vi "Begin.vi"(11 "Image Size":T1=enum."160x120") -> (0 "error out":errorcluster)   [LabVIEW 2011]
doc: "Called before other user functions, this VI is expected to open initial I/O refnums, load in file data, and do all program initialization. Notice that the <B>error out</B> terminal is simply used for data flow. Wiring it to other structures or subVIs ensures that this VI runs first."
uses:
  <vilib>/Rock Robotics/WPI/Camera/WPI_CameraImageSize.ctl
  <vilib>/Rock Robotics/WPI/Joystick/WPI_JoystickDeviceEnum.ctl
  <vilib>/Rock Robotics/SystemInterfaces/DIO/FPGA_DIOPWMChannel.ctl
  <vilib>/Rock Robotics/WPI/RobotDrive/WPI_RobotDriveOpen4MotorWithJaguar.vi
  <vilib>/Rock Robotics/WPI/Camera/WPI_CameraWhite Balance Values.ctl
  <vilib>/Rock Robotics/WPI/Camera/WPI_CameraExposure Values.ctl
  <vilib>/Rock Robotics/WPI/Camera/WPI_CameraFrameRate.ctl
  <vilib>/Rock Robotics/WPI/Relay/WPI_RelayDirection.ctl
  <vilib>/Rock Robotics/SystemInterfaces/Typedef/FPGA_TypedefDigitalModule.ctl
  <vilib>/Rock Robotics/SystemInterfaces/DIO/FPGA_DIORelayChannel.ctl
  <vilib>/Rock Robotics/WPI/MotorControl/WPI_MotorControlOpen Victor.vi
  <vilib>/Rock Robotics/SystemInterfaces/DIO/FPGA_DIOChannel.ctl
  <vilib>/Rock Robotics/WPI/MotorControl/WPI_MotorControlOpen Jaguar.vi
  <vilib>/Rock Robotics/WPI/Counter/WPI_CounterDigitalInputToDigitalSource.vi
  <vilib>/Rock Robotics/WPI/Encoder/WPI_EncoderType.ctl
  <vilib>/Rock Robotics/SystemInterfaces/AI/FPGA_AIGyroChannel.ctl
  <vilib>/Rock Robotics/SystemInterfaces/AI/FPGA_AIChannel.ctl
  <vilib>/Rock Robotics/WPI/MotorControl/WPI_MotorControlOpenCANJaguar.vi
  <vilib>/Rock Robotics/WPI/CAN/Jaguar/SubVIs/WPI_CANJaguar_ControlMode.ctl
  <vilib>/Rock Robotics/WPI/CAN/Jaguar/SubVIs/WPI_CANJaguar_SpeedReference.ctl
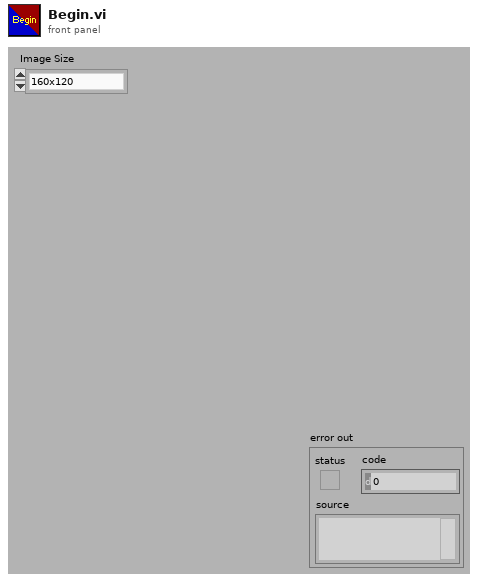
[diagram p1: front panel]
types:
  T1 = typedef "WPI_CameraImageSize.ctl" = enum16{"640x480", "320x240", "160x120"}
  T2 = typedef "FPGA_DIOPWMChannel.ctl" = enum8{"PWM 1", "PWM 2", "PWM 3", "PWM 4", "PWM 5", "PWM 6", "PWM 7", "PWM 8", "PWM 9", "PWM 10", "Invalid"}
  T3 = typedef "WPI_JoystickDeviceEnum.ctl" = enum16{"USB 1", "USB 2", "USB 3", "USB 4", "Kinect 1", "Kinect 2"}
  T4 = typedef "WPI_CameraFrameRate.ctl" = u32
  T5 = typedef "WPI_CameraExposure Values.ctl" = enum16{"Auto", "Flicker-free 50 Hz", "Flicker-free 60 Hz", "Hold current"}
  T6 = typedef "WPI_CameraWhite Balance Values.ctl" = enum16{"Auto", "Fixed indoor", "Fixed outdoor 1", "Fixed outdoor 2", "Fixed fluorescent 1", "Fixed fluorescent 2", "Hold current"}
  T7 = typedef "WPI_CameraDevRef.ctl" = cluster{"Camera Address":string, "CameraStatus":errorcluster, "Acquire Image Notifier":refnum<notifier>}
  T8 = typedef "FPGA_AIGyroChannel.ctl" = enum8{"AI 1", "AI 2", "Invalid"}
  T9 = typedef "WPI_GyroDevRef.ctl" = cluster{"DevStatus":errorcluster, "Analog Module":T10, "Analog Channel":T11, "Offset":dbl, "Gain (VoltsPerDegree/Second)":dbl}
  T10 = typedef "FPGA_TypedefAnalogModule.ctl" = enum16{"Analog Module 1", "Analog Module 2"}
  T11 = typedef "FPGA_AIChannel.ctl" = enum8{"AI 1", "AI 2", "AI 3", "AI 4", "AI 5", "AI 6", "AI 7", "AI 8", "Invalid"}
  T12 = typedef "FPGA_TypedefDigitalModule.ctl" = enum16{"Digital Module 1", "Digital Module 2"}
  T13 = typedef "WPI_CANJaguar_ControlMode.ctl" = enum8{"Percent VBus", "Current", "Speed", "Position", "Voltage"}
  T14 = typedef "WPI_MotorControlDeviceRef.ctl" = cluster{"DeviceStatus":errorcluster, "Type":enum16{"PWM", "CAN"}, "PWM":cluster{"Digital Module":T12, "PWM Channel":T2, "DeadBand":T15}, "CAN":cluster{"Device Number":u8, "Control Mode":T13, "Semaphore":T16, "Max Vout":dbl}, "Invert":bool, "TransformRef":T17, "InvTransformRef":T17}
  T15 = typedef "WPI_PWMDeadband.ctl" = cluster{"Name":string, "maxPositivePwm":i32, "minPositivePwm":i32, "centerPwm":i32, "maxNegativePwm":i32, "minNegativePwm":i32, "angularRange":u16}
  T16 = typedef "Semaphore RefNum" = refnum<k1>
  T17 = typedef "WPI_PWMTransform_ConPane.ctl" = refnum<vi>
  T18 = typedef "WPI_CANJaguar_SpeedReference.ctl" = u8
  T19 = typedef "FPGA_DIOChannel.ctl" = enum8{"DIO 1", "DIO 2", "DIO 3", "DIO 4", "DIO 5", "DIO 6", "DIO 7", "DIO 8", "DIO 9", "DIO 10", "DIO 11", "DIO 12", "DIO 13", "DIO 14", "Invalid"}
  T20 = typedef "WPI_DigitalInputDevRef.ctl" = cluster{"DevStatus":errorcluster, "DIO Channel":T19, "Digital Module":T12}
  T21 = typedef "WPI_EncoderType.ctl" = enum16{"1x", "2x", "4x"}
  T22 = typedef "FPGA_CounterEncoderSourceConvertionLVSourceType.ctl" = cluster{"DevStatus":errorcluster, "AnalogTriggerMode?":bool, "DigitalMode":cluster{"Digital Module":T12, "DIO Channel":T23}, "AnalogTriggerMode":cluster{"AnalogTriggerIndex":T24, "OutputType":T25}}
  T23 = typedef "FPGA_DIODigitalSourceChannel.ctl" = enum8{"DIO 1", "DIO 2", "DIO 3", "DIO 4", "DIO 5", "DIO 6", "DIO 7", "DIO 8", "DIO 9", "DIO 10", "DIO 11", "DIO 12", "DIO 13", "DIO 14", "Disabled"}
  T24 = typedef "FPGA_AnalogTriggerIndex.ctl" = enum8{"Trig 0", "Trig 1", "Trig 2", "Trig 3", "Trig 4", "Trig 5", "Trig 6", "Trig 7", "Invalid"}
  T25 = typedef "FPGA_AnalogTriggerOutType.ctl" = enum16{"InWindow", "TriggerState", "Rising", "Falling"}
  T26 = typedef "WPI_EncoderDevRef.ctl" = cluster{"DevStatus":errorcluster, "EncoderIndex":T27, "CounterIndex":T28, "DistancePerCount":dbl, "Decoding Type":T21}
  T27 = typedef "FPGA_EncoderIdx.ctl" = enum8{"Enc 0", "Enc 1", "Enc 2", "Enc 3", "Invalid"}
  T28 = typedef "FPGA_CounterCtrSystemIndex.ctl" = enum8{"Ctr 0", "Ctr 1", "Ctr 2", "Ctr 3", "Ctr 4", "Ctr 5", "Ctr 6", "Ctr 7", "Invalid"}
  T29 = typedef "WPI_ServoDeviceRef.ctl" = cluster{"DeviceStatus":errorcluster, "Digital Module":T12, "PWM Channel":T2, "DeadBand":T15}
  T30 = typedef "WPI_AnalogChannelDevRef.ctl" = cluster{"DevStatus":errorcluster, "Analog Module":T10, "Analog Channel":T11}
  T31 = typedef "FPGA_DIORelayChannel.ctl" = enum8{"Relay 1", "Relay 2", "Relay 3", "Relay 4", "Relay 5", "Relay 6", "Relay 7", "Relay 8", "Invalid"}
  T32 = typedef "WPI_RelayDirection.ctl" = enum16{"Both directions", "Forward only", "Reverse only"}
  T33 = typedef "WPI_RelayDevRef.ctl" = cluster{"DevStatus":errorcluster, "Relay Channel":T31, "Digital Module":T12, "Relay Direction":T32}
  T34 = typedef "WPI_RobotDriveDevRef.ctl" = cluster{"DevStatus":errorcluster, "Motors[]":T14[], "Square Inputs":bool, "Max Output":dbl, "Isochronous":bool}
  T35 = typedef "WPI_JoystickDevRef.ctl" = cluster{"Device":T3}
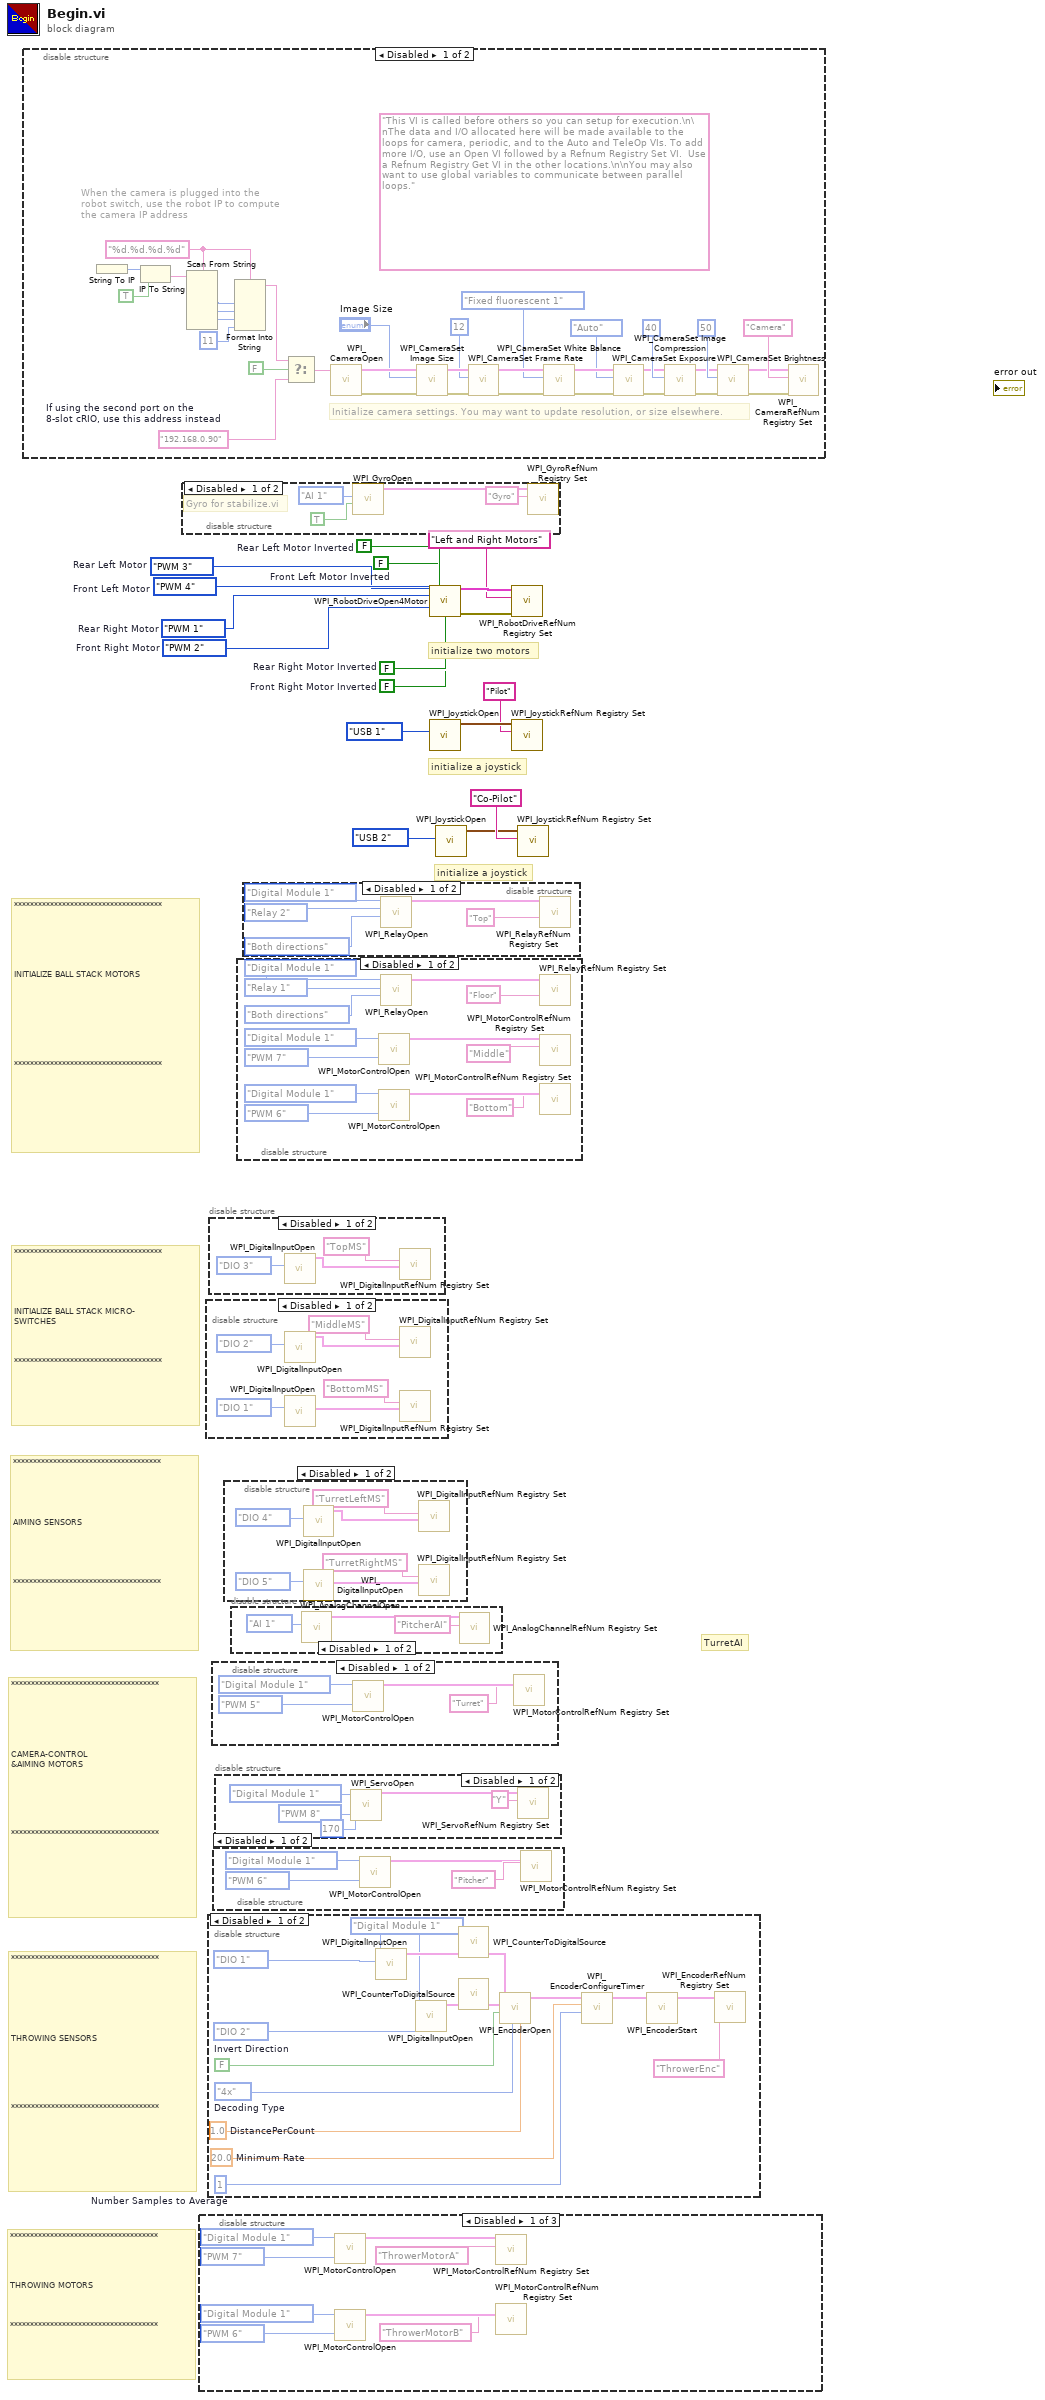
[diagram p0: block diagram]
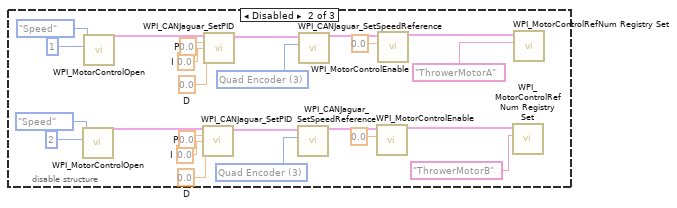
[diagram p13: hidden frame]
diagram:
  w1 = FALSE  # Front Right Motor Inverted
  w2 = FALSE  # Front Left Motor Inverted
  w3 = FPGA_DIOPWMChannel."PWM 3"  # Rear Left Motor
  w4 = FPGA_DIOPWMChannel."PWM 1"  # Rear Right Motor
  w5 = FPGA_DIOPWMChannel."PWM 2"  # Front Right Motor
  w6 = FPGA_DIOPWMChannel."PWM 4"  # Front Left Motor
  w16 = FALSE  # Rear Left Motor Inverted
  w17 = FALSE  # Rear Right Motor Inverted
  # "TurretAI"
  # "*************************************\n\n\n\n\nTHROWING MOTORS\n\n\n\n*************************************"
  # "*************************************\n\n\n\n\n\n\n\nTHROWING SENSORS\n\n\n\n\n\n\n*************************************"
  # "*************************************\n\n\n\n\n\n\nCAMERA-CONTROL\n&AIMING MOTORS\n\n\n\n\n\n\n*************************************"
  # "*************************************\n\n\n\n\n\nAIMING SENSORS\n\n\n\n\n\n*************************************"
  # "*************************************\n\n\n\n\n\nINITIALIZE BALL STACK MICRO-\nSWITCHES\n\n\n\n*************************************"
  # "*************************************\n\n\n\n\n\n\nINITIALIZE BALL STACK MOTORS\n\n\n\n\n\n\n\n\n*************************************"
  # "initialize a joystick"
  # "initialize a joystick"
  # "initialize two motors"
  n1 = disable-structure shown="Disabled" {
    frame Disabled {
      w22 = "%d.%d.%d.%d" ("format string")
      (unwired) "This VI is called before others so you can setup for execution.\n\nThe data and I/O allocated here will be made available to the loops for camera, periodic, and to the Auto and TeleOp VIs. To add more I/O, use an Open VI followed by a Refnum Registry Set VI.  Use a Refnum Registry Get VI in the other locations.\n\nYou may also want to use global variables to communicate between parallel loops."
      w19 = "192.168.0.90"  # If using the second port on the 8-slot cRIO, use this address instead
      # "When the camera is plugged into the\nrobot switch, use the robot IP to compute\nthe camera IP address"
      # "Initialize camera settings. You may want to update resolution, or size elsewhere."
      n2 = String To IP() -> (0:w29:u32)  [unwired: 1 in]
      n3 = IP To String(1:TRUE ("dot notation? (F)"), 2:w29) -> (0:w27:string)
      n4 = Scan From String(format string=w22, input string=w27) -> (output 1=w26:i32, output 2=w25:i32, output 3=w24:i32)  [unwired: 7 in, 3 out]
      n5 = Format Into String(format string=w22, w26, w25, w24, 11 ("Compression")) -> (resulting string=w20:string)  [unwired: 2 in, 1 out]
      n6 = Select(t=w20, s=FALSE, f=w19) -> (s? t:f=w21:string)
      n7 = call <vilib>:"WPI_CameraOpen.vi"("Camera Address"=w21) -> ("error out"=w41:errorcluster, "CameraDevRef"=w42:T7)  [unwired: 1 in, 8 out]
      n8 = call <vilib>:"WPI_CameraSet Image Size.vi"("error in (no error)"=w41, "Image Size"="Image Size", "CameraDevRef"=w42) -> ("error out"=w40:errorcluster, "CameraDevRef Out"=w43:T7)  [unwired: 7 out]
      n9 = call <vilib>:"WPI_CameraSet Frame Rate.vi"("error in (no error)"=w40, "Frame Rate (fps)"=T4 12, "CameraDevRef"=w43) -> ("error out"=w39:errorcluster, "CameraDevRef Out"=w45:T7)  [unwired: 7 out]
      n10 = call <vilib>:"WPI_CameraSet White Balance.vi"("error in (no error)"=w39, "White Balance"=WPI_CameraWhite_Balance_Values."Fixed fluorescent 1", "CameraDevRef"=w45) -> ("error out"=w38:errorcluster, "CameraDevRef Out"=w44:T7)  [unwired: 7 out]
      n11 = call <vilib>:"WPI_CameraSet Exposure.vi"("error in (no error)"=w38, "Exposure"=WPI_CameraExposure_Values."Auto", "CameraDevRef"=w44) -> ("error out"=w37:errorcluster, "CameraDevRef Out"=w47:T7)  [unwired: 7 out]
      n12 = call <vilib>:"WPI_CameraSet Image Compression.vi"("error in (no error)"=w37, "Compression"=40, "CameraDevRef"=w47) -> ("error out"=w36:errorcluster, "CameraDevRef Out"=w46:T7)  [unwired: 7 out]
      n13 = call <vilib>:"WPI_CameraSet Brightness.vi"("error in (no error)"=w36, "Brightness"=50, "CameraDevRef"=w46) -> ("error out"=w34:errorcluster, "CameraDevRef Out"=w35:T7)  [unwired: 7 out]
      n14 = call <vilib>:"WPI_CameraRefNum Registry Set.vi"("error in (no error)"=w34, "refnum name"="Camera", "CameraDevRef"=w35) -> ()  [unwired: 9 out]
    }
    frame Enabled {
    }
  }
  n15 = disable-structure shown="Disabled" {
    frame Disabled {
      # "Gyro for stabilize.vi"
      n16 = call <vilib>:"WPI_GyroOpen.vi"("Calibrate On Open"=TRUE, "Analog Channel"=FPGA_AIGyroChannel."AI 1") -> ("GyroDevRef"=w54:T9)  [unwired: 7 in, 2 out]
      n17 = call <vilib>:"WPI_GyroRefNum Registry Set.vi"("refnum name"="Gyro", "GyroDevRef"=w54) -> ()  [unwired: 8 in, 2 out]
    }
    frame Enabled {
    }
  }
  n18 = disable-structure shown="Disabled" {
    frame Disabled {
      n19 = call-poly <vilib>:"WPI_MotorControlOpen.vi"("PWM Channel"=FPGA_DIOPWMChannel."PWM 7", "Digital Module (Module 1)"=FPGA_TypedefDigitalModule."Digital Module 1") -> ("MotorControlDeviceRef"=w62:T14)  [unwired: 8 in, 1 out]
      n20 = call-poly <vilib>:"WPI_MotorControlOpen.vi"("PWM Channel"=FPGA_DIOPWMChannel."PWM 6", "Digital Module (Module 1)"=FPGA_TypedefDigitalModule."Digital Module 1") -> ("MotorControlDeviceRef"=w58:T14)  [unwired: 8 in, 1 out]
      n21 = call <vilib>:"WPI_MotorControlRefNum Registry Set.vi"("refnum name"="ThrowerMotorA", "MotorControlDevRef"=w62) -> ()  [unwired: 8 in, 2 out]
      n22 = call <vilib>:"WPI_MotorControlRefNum Registry Set.vi"("refnum name"="ThrowerMotorB", "MotorControlDevRef"=w58) -> ()  [unwired: 8 in, 2 out]
    }
    frame Disabled {
      w75 = 0.0  # D
      w74 = 0.0  # I
      w73 = 0.0  # P
      w70 = T18 3 items=["Encoder"=0, "Inv Encoder"=2, "Quad Encoder"=3, "None"=255] ("Speed Reference")
      w76 = 0.0  # D
      w77 = 0.0  # I
      w78 = 0.0  # P
      w81 = T18 3 items=["Encoder"=0, "Inv Encoder"=2, "Quad Encoder"=3, "None"=255] ("Speed Reference")
      n23 = call-poly <vilib>:"WPI_MotorControlOpen.vi"("Device Number"=u8 2, "Control Mode"=WPI_CANJaguar_ControlMode."Speed") -> ("MotorControlDeviceRef"=w71:T14)  [unwired: 8 in, 1 out]
      n24 = call-poly <vilib>:"WPI_MotorControlOpen.vi"("Device Number"=u8 1, "Control Mode"=WPI_CANJaguar_ControlMode."Speed") -> ("MotorControlDeviceRef"=w80:T14)  [unwired: 8 in, 1 out]
      n25 = call <vilib>:"WPI_CANJaguar_SetPID.vi"("CAN Jaguar Ref"=w71, "P"=w73, "I"=w74, "D"=w75) -> ("CAN Jaguar Ref Out"=w69:T14)  [unwired: 10 in, 1 out]
      n26 = call <vilib>:"WPI_CANJaguar_SetPID.vi"("CAN Jaguar Ref"=w80, "P"=w78, "I"=w77, "D"=w76) -> ("CAN Jaguar Ref Out"=w82:T14)  [unwired: 10 in, 1 out]
      n27 = call <vilib>:"WPI_CANJaguar_SetSpeedReference.vi"("Speed Reference"=w70, "CAN Jaguar Ref"=w69) -> ("CAN Jaguar Ref Out"=w67:T14)  [unwired: 8 in, 1 out]
      n28 = call <vilib>:"WPI_CANJaguar_SetSpeedReference.vi"("Speed Reference"=w81, "CAN Jaguar Ref"=w82) -> ("CAN Jaguar Ref Out"=w84:T14)  [unwired: 8 in, 1 out]
      n29 = call <vilib>:"WPI_MotorControlEnable.vi"("Encoder Initial Position"=0.0, "CAN Jaguar Ref"=w67) -> ("CAN Jaguar Ref Out"=w66:T14)  [unwired: 8 in, 1 out]
      n30 = call <vilib>:"WPI_MotorControlEnable.vi"("Encoder Initial Position"=0.0, "CAN Jaguar Ref"=w84) -> ("CAN Jaguar Ref Out"=w85:T14)  [unwired: 8 in, 1 out]
      n31 = call <vilib>:"WPI_MotorControlRefNum Registry Set.vi"("refnum name"="ThrowerMotorB", "MotorControlDevRef"=w66) -> ()  [unwired: 8 in, 2 out]
      n32 = call <vilib>:"WPI_MotorControlRefNum Registry Set.vi"("refnum name"="ThrowerMotorA", "MotorControlDevRef"=w85) -> ()  [unwired: 8 in, 2 out]
    }
    frame Enabled {
    }
  }
  n33 = disable-structure shown="Disabled" {
    frame Disabled {
      n34 = call <vilib>:"WPI_DigitalInputOpen.vi"("DIO Channel"=FPGA_DIOChannel."DIO 2") -> ("DigitalInputDevRef"=w87:T20)  [unwired: 9 in, 1 out]
      n35 = call <vilib>:"WPI_DigitalInputOpen.vi"("DIO Channel"=FPGA_DIOChannel."DIO 1") -> ("DigitalInputDevRef"=w90:T20)  [unwired: 9 in, 1 out]
      n36 = call <vilib>:"WPI_DigitalInputRefNum Registry Set.vi"("refnum name"="MiddleMS", "DigitalInputDevRef"=w87) -> ()  [unwired: 8 in, 2 out]
      n37 = call <vilib>:"WPI_DigitalInputRefNum Registry Set.vi"("refnum name"="BottomMS", "DigitalInputDevRef"=w90) -> ()  [unwired: 8 in, 2 out]
    }
    frame Enabled {
    }
  }
  n38 = disable-structure shown="Disabled" {
    frame Disabled {
      w96 = u8 1  # Number Samples to Average
      w97 = 20.0  # Minimum Rate
      w102 = 1.0  # DistancePerCount
      w101 = WPI_EncoderType."4x"  # Decoding Type
      w100 = FALSE  # Invert Direction
      w95 = FPGA_TypedefDigitalModule."Digital Module 1" ("DIO Module")
      n39 = call <vilib>:"WPI_DigitalInputOpen.vi"("DIO Channel"=FPGA_DIOChannel."DIO 1" ("A Channel"), "Digital Module (Module 1)"=w95) -> ("DigitalInputDevRef"=w106:T20)  [unwired: 1 in, 8 out]
      n40 = call <vilib>:"WPI_DigitalInputOpen.vi"("DIO Channel"=FPGA_DIOChannel."DIO 2" ("B Channel"), "Digital Module (Module 1)"=w95) -> ("DigitalInputDevRef"=w107:T20)  [unwired: 1 in, 8 out]
      n41 = call-poly <vilib>:"WPI_CounterToDigitalSource.vi"("DigitalInputDevRef"=w106) -> ("Digital Source"=w105:T22)  [unwired: 6 out]
      n42 = call-poly <vilib>:"WPI_CounterToDigitalSource.vi"("DigitalInputDevRef"=w107) -> ("Digital Source"=w108:T22)  [unwired: 6 out]
      n43 = call <vilib>:"WPI_EncoderOpen.vi"("DistancePerCount"=w102, "Decoding Type"=w101, "Invert Direction (False)"=w100, "BSource"=w108, "ASource"=w105) -> ("EncoderDevRef"=w98:T26)  [unwired: 3 in, 3 out]
      n44 = call <vilib>:"WPI_EncoderConfigureTimer.vi"("Number Samples to Average"=w96, "Minimum Rate"=w97, "EncoderDevRef"=w98) -> ("EncoderDevRef"=w99:T26)  [unwired: 1 in, 7 out]
      n45 = call <vilib>:"WPI_EncoderStart.vi"("EncoderDevRef"=w99) -> ("EncoderDevRef"=w94:T26)  [unwired: 1 in, 9 out]
      n46 = call <vilib>:"WPI_EncoderRefNum Registry Set.vi"("refnum name"="ThrowerEnc", "EncoderDevRef"=w94) -> ()  [unwired: 8 in, 2 out]
    }
    frame Enabled {
    }
  }
  n47 = disable-structure shown="Disabled" {
    frame Disabled {
      n48 = call <vilib>:"WPI_DigitalInputOpen.vi"("DIO Channel"=FPGA_DIOChannel."DIO 3") -> ("DigitalInputDevRef"=w111:T20)  [unwired: 9 in, 1 out]
      n49 = call <vilib>:"WPI_DigitalInputRefNum Registry Set.vi"("refnum name"="TopMS", "DigitalInputDevRef"=w111) -> ()  [unwired: 8 in, 2 out]
    }
    frame Enabled {
    }
  }
  n50 = disable-structure shown="Disabled" {
    frame Disabled {
      n51 = call-poly <vilib>:"WPI_MotorControlOpen.vi"("PWM Channel"=FPGA_DIOPWMChannel."PWM 5", "Digital Module (Module 1)"=FPGA_TypedefDigitalModule."Digital Module 1") -> ("MotorControlDeviceRef"=w115:T14)  [unwired: 8 in, 1 out]
      n52 = call <vilib>:"WPI_MotorControlRefNum Registry Set.vi"("refnum name"="Turret", "MotorControlDevRef"=w115) -> ()  [unwired: 8 in, 2 out]
    }
    frame Enabled {
    }
  }
  n53 = disable-structure shown="Disabled" {
    frame Disabled {
      n54 = call-poly <vilib>:"WPI_MotorControlOpen.vi"("PWM Channel"=FPGA_DIOPWMChannel."PWM 6", "Digital Module (Module 1)"=FPGA_TypedefDigitalModule."Digital Module 1") -> ("MotorControlDeviceRef"=w116:T14)  [unwired: 8 in, 1 out]
      n55 = call <vilib>:"WPI_MotorControlRefNum Registry Set.vi"("refnum name"="Pitcher", "MotorControlDevRef"=w116) -> ()  [unwired: 8 in, 2 out]
    }
    frame Enabled {
    }
  }
  n56 = disable-structure shown="Disabled" {
    frame Disabled {
      n57 = call <vilib>:"WPI_ServoOpen.vi"("Angular Range"=u16 170, "PWM Channel"=FPGA_DIOPWMChannel."PWM 8", "Digital Module (Module 1)"=FPGA_TypedefDigitalModule."Digital Module 1") -> ("ServoDeviceRef"=w121:T29)  [unwired: 7 in, 1 out]
      n58 = call <vilib>:"WPI_ServoRefNum Registry Set.vi"("refnum name"="Y", "ServoDeviceRef"=w121) -> ()  [unwired: 8 in, 2 out]
    }
    frame Enabled {
    }
  }
  n59 = disable-structure shown="Disabled" {
    frame Disabled {
      n60 = call <vilib>:"WPI_DigitalInputOpen.vi"("DIO Channel"=FPGA_DIOChannel."DIO 4") -> ("DigitalInputDevRef"=w125:T20)  [unwired: 9 in, 1 out]
      n61 = call <vilib>:"WPI_DigitalInputOpen.vi"("DIO Channel"=FPGA_DIOChannel."DIO 5") -> ("DigitalInputDevRef"=w128:T20)  [unwired: 9 in, 1 out]
      n62 = call <vilib>:"WPI_DigitalInputRefNum Registry Set.vi"("refnum name"="TurretLeftMS", "DigitalInputDevRef"=w125) -> ()  [unwired: 8 in, 2 out]
      n63 = call <vilib>:"WPI_DigitalInputRefNum Registry Set.vi"("refnum name"="TurretRightMS", "DigitalInputDevRef"=w128) -> ()  [unwired: 8 in, 2 out]
    }
    frame Enabled {
    }
  }
  n64 = disable-structure shown="Disabled" {
    frame Disabled {
      n65 = call <vilib>:"WPI_AnalogChannelOpen.vi"("Analog Channel"=FPGA_AIChannel."AI 1") -> ("AIDeviceRef"=w133:T30)  [unwired: 9 in, 1 out]
      n66 = call <vilib>:"WPI_AnalogChannelRefNum Registry Set.vi"("refnum name"="PitcherAI", "AIDeviceRef"=w133) -> ()  [unwired: 8 in, 2 out]
    }
    frame Enabled {
    }
  }
  n67 = disable-structure shown="Disabled" {
    frame Disabled {
      n68 = call-poly <vilib>:"WPI_MotorControlOpen.vi"("PWM Channel"=FPGA_DIOPWMChannel."PWM 7", "Digital Module (Module 1)"=FPGA_TypedefDigitalModule."Digital Module 1") -> ("MotorControlDeviceRef"=w141:T14)  [unwired: 8 in, 1 out]
      n69 = call-poly <vilib>:"WPI_MotorControlOpen.vi"("PWM Channel"=FPGA_DIOPWMChannel."PWM 6", "Digital Module (Module 1)"=FPGA_TypedefDigitalModule."Digital Module 1") -> ("MotorControlDeviceRef"=w137:T14)  [unwired: 8 in, 1 out]
      n70 = call <vilib>:"WPI_RelayOpen.vi"("Relay Direction"=WPI_RelayDirection."Both directions", "Relay Channel"=FPGA_DIORelayChannel."Relay 1", "Digital Module (Module 1)"=FPGA_TypedefDigitalModule."Digital Module 1") -> ("RelayDevRef"=w143:T33)  [unwired: 7 in, 1 out]
      n71 = call <vilib>:"WPI_RelayRefNum Registry Set.vi"("refnum name"="Floor", "RelayDevRef"=w143) -> ()  [unwired: 8 in, 2 out]
      n72 = call <vilib>:"WPI_MotorControlRefNum Registry Set.vi"("refnum name"="Middle", "MotorControlDevRef"=w141) -> ()  [unwired: 8 in, 2 out]
      n73 = call <vilib>:"WPI_MotorControlRefNum Registry Set.vi"("refnum name"="Bottom", "MotorControlDevRef"=w137) -> ()  [unwired: 8 in, 2 out]
    }
    frame Enabled {
    }
  }
  n74 = disable-structure shown="Disabled" {
    frame Disabled {
      n75 = call <vilib>:"WPI_RelayOpen.vi"("Relay Direction"=WPI_RelayDirection."Both directions", "Relay Channel"=FPGA_DIORelayChannel."Relay 2", "Digital Module (Module 1)"=FPGA_TypedefDigitalModule."Digital Module 1") -> ("RelayDevRef"=w150:T33)  [unwired: 7 in, 1 out]
      n76 = call <vilib>:"WPI_RelayRefNum Registry Set.vi"("refnum name"="Top", "RelayDevRef"=w150) -> ()  [unwired: 8 in, 2 out]
    }
    frame Enabled {
    }
  }
  n77 = call-poly <vilib>:"WPI_RobotDriveOpen4Motor.vi"("Rear Left Motor"=w3, "Rear Left Motor Inverted"=w16, "Rear Right Motor Inverted"=w17, "Rear Right Motor"=w4, "Front Left Motor"=w6, "Front Right Motor"=w5, "Front Left Motor Inverted"=w2, "Front Right Motor Inverted"=w1) -> ("RobotDriveDevRef"=w15:T34, "error out"=w11:errorcluster)  [unwired: 6 in]
  n78 = call <vilib>:"WPI_JoystickOpen.vi"("JoystickDevice"=WPI_JoystickDeviceEnum."USB 1") -> ("JoystickDevRef"=w13:T35)  [unwired: 10 out]
  n79 = call <vilib>:"WPI_JoystickOpen.vi"("JoystickDevice"=WPI_JoystickDeviceEnum."USB 2") -> ("JoystickDevRef"=w7:T35)  [unwired: 10 out]
  n80 = call <vilib>:"WPI_RobotDriveRefNum Registry Set.vi"("error in (no error)"=w11, "refnum name"="Left and Right Motors", "RobotDriveDevRef"=w15) -> ()  [unwired: 9 out]
  n81 = call <vilib>:"WPI_JoystickRefNum Registry Set.vi"("refnum name"="Pilot", "JoystickDevRef"=w13) -> ()  [unwired: 1 in, 9 out]
  n82 = call <vilib>:"WPI_JoystickRefNum Registry Set.vi"("refnum name"="Co-Pilot", "JoystickDevRef"=w7) -> ()  [unwired: 1 in, 9 out]
